vi "DAQPXInameToSlotNumber.vi"(1 "PXI name":string="PXI_Star2") -> (0 "Slot #":string)   [LabVIEW 2014]
doc: "Grabs the slot number from the NI physical name, and outputs it as a string for storage."
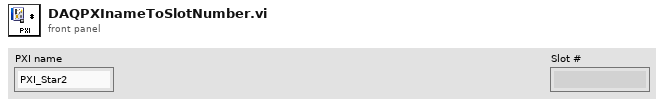
[diagram p1: front panel]
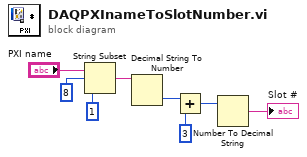
[diagram p0: block diagram]
diagram:
  n1 = String Subset(string="PXI name", offset (0)=8, length (rest)=1 ("length (rest)")) -> (substring=w5:string)
  n2 = Decimal String To Number(string=w5) -> (number=w4:i32)  [unwired: 2 in, 1 out]
  n3 = Add(x=w4, y=3) -> (x+y=w2:i32)
  n4 = Number To Decimal String(number=w2) -> (decimal integer string=→"Slot #":string)  [unwired: 1 in]
